vi "Read File.vi"(8 "error in (no error)":errorcluster, 11 "TDMS Properties in":refnum<class "TDMS Properties.lvclass">) -> (0 "error out":errorcluster, 2 "File":path, 3 "TDMS Properties out":refnum<class "TDMS Properties.lvclass">)   [LabVIEW 2019, in "TDMS Properties.lvclass"]
uses:
  TDMS Properties.lvclass
  TDMS Properties.lvclass/TDMS Properties.ctl
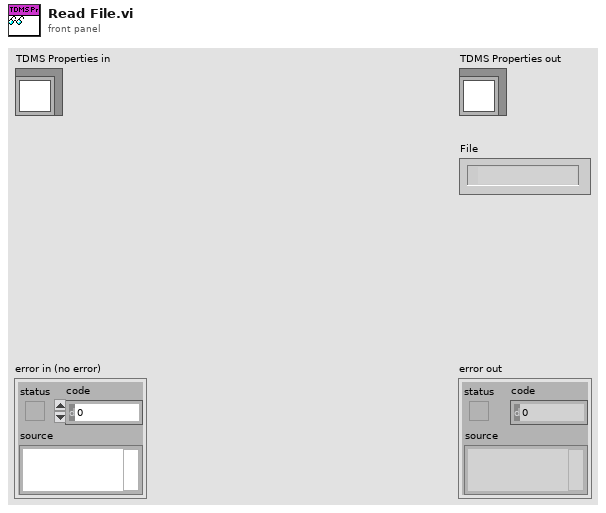
[diagram p1: front panel]
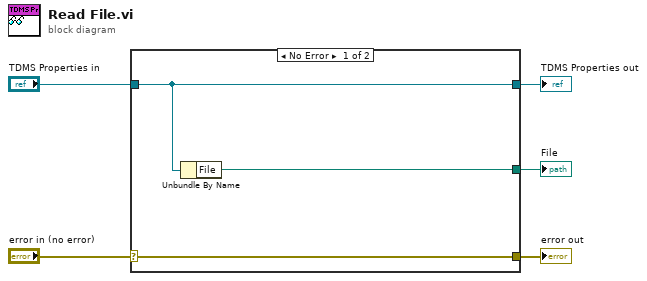
[diagram p0: block diagram]
diagram:
  n1 = case shown="No Error" "error in (no error)" {
    selector: "error in (no error)" -> [w8 w9]
    tunnel: [w8 w9] -> w4
    tunnel: [w7 w10] -> w2
    tunnel: "TDMS Properties in" -> [w7 w10]
    tunnel: [w6 _] -> w1
    frame No Error {
      n2 = Unbundle By Name(w7) -> ("File"=w6:path)
    }
    frame Error {
    }
  }
  "error out" <- w4
  "TDMS Properties out" <- w2
  "File" <- w1
